vi "niWLAN - 80211abgnGeneration.vi"(0 "Rx Measurements Settings":T1={"Standard"=3, "Channel Bandwidth (Hz)"=40000000.0, "Idle Interval (s)"=400000.0, "MCS Index"=7, "80211n PLCP Frame Format"=0, "Payload Data Length (bytes)"=1024, "OFDM Data Rate (Mbps)"=0, "DSSS Data Rate (Mbps)"=0, "HW Settings"=[{"Carrier Frequency(Hz)"=5190000000.0, "power Level(dBm)"=[-10.0, -12.0, -14.0, -16.0, -18.0, -20.0, -22.0, -24.0, -26.0, -28.0, -30.0, -32.0, -34.0, -36.0, -38.0, -40.0, -42.0, -44.0, -46.0, -48.0, -50.0, -52.0, -54.0, -56.0, -58.0, -60.0, -62.0, -64.0, -66.0, -68.0, -70.0, -72.0, -74.0, -76.0, -78.0, -80.0, -82.0, -84.0], "power Level(milli-dBm)"=[-10000, -12000, -14000, -16000, -18000, -20000, -22000, -24000, -26000, -28000, -30000, -32000, -34000, -36000, -38000, -40000, -42000, -44000, -46000, -48000, -50000, -52000, -54000, -56000, -58000, -60000, -62000, -64000, -66000, -68000, -70000, -72000, -74000, -76000, -78000, -80000, -82000, -84000]}, {"Carrier Frequency(Hz)"=5230000000.0, "power Level(dBm)"=[-10.0, -12.0, -14.0, -16.0, -18.0, -20.0, -22.0, -24.0, -26.0, -28.0, -30.0, -32.0, -34.0, -36.0, -38.0, -40.0, -42.0, -44.0, -46.0, -48.0, -50.0, -52.0, -54.0, -56.0, -58.0, -60.0, -62.0, -64.0, -66.0, -68.0, -70.0, -72.0, -74.0, -76.0, -78.0, -80.0, -82.0, -84.0], "power Level(milli-dBm)"=[-10000, -12000, -14000, -16000, -18000, -20000, -22000, -24000, -26000, -28000, -30000, -32000, -34000, -36000, -38000, -40000, -42000, -44000, -46000, -48000, -50000, -52000, -54000, -56000, -58000, -60000, -62000, -64000, -66000, -68000, -70000, -72000, -74000, -76000, -78000, -80000, -82000, -84000]}, {"Carrier Frequency(Hz)"=5310000000.0, "power Level(dBm)"=[-10.0, -12.0, -14.0, -16.0, -18.0, -20.0, -22.0, -24.0, -26.0, -28.0, -30.0, -32.0, -34.0, -36.0, -38.0, -40.0, -42.0, -44.0, -46.0, -48.0, -50.0, -52.0, -54.0, -56.0, -58.0, -60.0, -62.0, -64.0, -66.0, -68.0, -70.0, -72.0, -74.0, -76.0, -78.0, -80.0, -82.0, -84.0], "power Level(milli-dBm)"=[-10000, -12000, -14000, -16000, -18000, -20000, -22000, -24000, -26000, -28000, -30000, -32000, -34000, -36000, -38000, -40000, -42000, -44000, -46000, -48000, -50000, -52000, -54000, -56000, -58000, -60000, -62000, -64000, -66000, -68000, -70000, -72000, -74000, -76000, -78000, -80000, -82000, -84000]}, {"Carrier Frequency(Hz)"=5510000000.0, "power Level(dBm)"=[-10.0, -12.0, -14.0, -16.0, -18.0, -20.0, -22.0, -24.0, -26.0, -28.0, -30.0, -32.0, -34.0, -36.0, -38.0, -40.0, -42.0, -44.0, -46.0, -48.0, -50.0, -52.0, -54.0, -56.0, -58.0, -60.0, -62.0, -64.0, -66.0, -68.0, -70.0, -72.0, -74.0, -76.0, -78.0, -80.0, -82.0, -84.0], "power Level(milli-dBm)"=[-10000, -12000, -14000, -16000, -18000, -20000, -22000, -24000, -26000, -28000, -30000, -32000, -34000, -36000, -38000, -40000, -42000, -44000, -46000, -48000, -50000, -52000, -54000, -56000, -58000, -60000, -62000, -64000, -66000, -68000, -70000, -72000, -74000, -76000, -78000, -80000, -82000, -84000]}, {"Carrier Frequency(Hz)"=5630000000.0, "power Level(dBm)"=[-10.0, -12.0, -14.0, -16.0, -18.0, -20.0, -22.0, -24.0, -26.0, -28.0, -30.0, -32.0, -34.0, -36.0, -38.0, -40.0, -42.0, -44.0, -46.0, -48.0, -50.0, -52.0, -54.0, -56.0, -58.0, -60.0, -62.0, -64.0, -66.0, -68.0, -70.0, -72.0, -74.0, -76.0, -78.0, -80.0, -82.0, -84.0], "power Level(milli-dBm)"=[-10000, -12000, -14000, -16000, -18000, -20000, -22000, -24000, -26000, -28000, -30000, -32000, -34000, -36000, -38000, -40000, -42000, -44000, -46000, -48000, -50000, -52000, -54000, -56000, -58000, -60000, -62000, -64000, -66000, -68000, -70000, -72000, -74000, -76000, -78000, -80000, -82000, -84000]}, {"Carrier Frequency(Hz)"=5670000000.0, "power Level(dBm)"=[-10.0, -12.0, -14.0, -16.0, -18.0, -20.0, -22.0, -24.0, -26.0, -28.0, -30.0, -32.0, -34.0, -36.0, -38.0, -40.0, -42.0, -44.0, -46.0, -48.0, -50.0, -52.0, -54.0, -56.0, -58.0, -60.0, -62.0, -64.0, -66.0, -68.0, -70.0, -72.0, -74.0, -76.0, -78.0, -80.0, -82.0, -84.0], "power Level(milli-dBm)"=[-10000, -12000, -14000, -16000, -18000, -20000, -22000, -24000, -26000, -28000, -30000, -32000, -34000, -36000, -38000, -40000, -42000, -44000, -46000, -48000, -50000, -52000, -54000, -56000, -58000, -60000, -62000, -64000, -66000, -68000, -70000, -72000, -74000, -76000, -78000, -80000, -82000, -84000]}, {"Carrier Frequency(Hz)"=5755000000.0, "power Level(dBm)"=[-10.0, -12.0, -14.0, -16.0, -18.0, -20.0, -22.0, -24.0, -26.0, -28.0, -30.0, -32.0, -34.0, -36.0, -38.0, -40.0, -42.0, -44.0, -46.0, -48.0, -50.0, -52.0, -54.0, -56.0, -58.0, -60.0, -62.0, -64.0, -66.0, -68.0, -70.0, -72.0, -74.0, -76.0, -78.0, -80.0, -82.0, -84.0], "power Level(milli-dBm)"=[-10000, -12000, -14000, -16000, -18000, -20000, -22000, -24000, -26000, -28000, -30000, -32000, -34000, -36000, -38000, -40000, -42000, -44000, -46000, -48000, -50000, -52000, -54000, -56000, -58000, -60000, -62000, -64000, -66000, -68000, -70000, -72000, -74000, -76000, -78000, -80000, -82000, -84000]}, {"Carrier Frequency(Hz)"=5795000000.0, "power Level(dBm)"=[-10.0, -12.0, -14.0, -16.0, -18.0, -20.0, -22.0, -24.0, -26.0, -28.0, -30.0, -32.0, -34.0, -36.0, -38.0, -40.0, -42.0, -44.0, -46.0, -48.0, -50.0, -52.0, -54.0, -56.0, -58.0, -60.0, -62.0, -64.0, -66.0, -68.0, -70.0, -72.0, -74.0, -76.0, -78.0, -80.0, -82.0, -84.0], "power Level(milli-dBm)"=[-10000, -12000, -14000, -16000, -18000, -20000, -22000, -24000, -26000, -28000, -30000, -32000, -34000, -36000, -38000, -40000, -42000, -44000, -46000, -48000, -50000, -52000, -54000, -56000, -58000, -60000, -62000, -64000, -66000, -68000, -70000, -72000, -74000, -76000, -78000, -80000, -82000, -84000]}]} {"DSSS Data Rate (Mbps)" items=["1", "2", "5.5 CCK", "5.5 PBCC", "11 CCK", "11 PBCC", "22", "33"]; "OFDM Data Rate (Mbps)" items=["6", "9", "12", "18", "24", "36", "48", "54"]; "80211n PLCP Frame Format" items=["Mixed Format", "Greenfield Format"]; "Standard" items=["80211A/G/J/P OFDM", "80211B/G DSSS", "80211G DSSSOFDM", "80211N MIMOOFDM", "80211AC MIMOOFDM"]}, 7 "Address String":string="00:90:4C:C5:12:38", 11 "error in":errorcluster={"status"=FALSE, "code"=373404, "source"="niRFSG Check Generation Status.vi<ERR>DSP overflow detected. Output waveform was clipped. Reduce the Arb Pre Filter Gain to eliminate overflow.\n\n "}) -> (4 "actual headroom (dB)":dbl, 6 "Waveforms":cluster{"t0":dbl, "dt":dbl, "Y":cdb[]}[](array[cluster])=[{"t0"=0.0, "dt"=1.25e-08, "Y"=[0.0+0.0i, 0.0+0.0i, 0.0+0.0i, 0.0+0.0i, 0.0+0.0i, 0.0+0.0i, 0.0+0.0i, 0.0+0.0i, 0.0+0.0i, 0.0+0.0i, 0.0+0.0i, 0.0+0.0i, 0.0+0.0i, 0.0+0.0i, 0.0+0.0i, 0.0+0.0i, 0.0+0.0i, 0.0+0.0i, 0.0+0.0i, 0.0+0.0i, 0.0+0.0i, 0.0+0.0i, 0.0+0.0i, 0.0+0.0i, 0.0+0.0i, 0.0+0.0i, 0.0+0.0i, 0.0+0.0i, 0.0+0.0i, 0.0+0.0i, 0.0+0.0i, 0.0+0.0i, 0.0+0.0i, 0.0+0.0i, 0.0+0.0i, 0.0+0.0i, 0.0+0.0i, 0.0+0.0i, 0.0+0.0i, 0.0+0.0i, 0.0+0.0i, 0.0+0.0i, 0.0+0.0i, 0.0+0.0i, 0.0+0.0i, 0.0+0.0i, 0.0+0.0i, 0.0+0.0i, 0.0+0.0i, 0.0+0.0i, 0.0+0.0i, 0.0+0.0i, 0.0+0.0i, 0.0+0.0i, 0.0+0.0i, 0.0+0.0i, 0.0+0.0i, 0.0+0.0i, 0.0+0.0i, 0.0+0.0i, 0.0+0.0i, 0.0+0.0i, 0.0+0.0i, 0.0+0.0i, 0.0+0.0i, 0.0+0.0i, 0.0+0.0i, 0.0+0.0i, 0.0+0.0i, 0.0+0.0i, 0.0+0.0i, 0.0+0.0i, 0.0+0.0i, 0.0+0.0i, 0.0+0.0i, 0.0+0.0i, 0.0+0.0i, 0.0+0.0i, 0.0+0.0i, 0.0+0.0i, 0.0+0.0i, 0.0+0.0i, 0.0+0.0i, 0.0+0.0i, 0.0+0.0i, 0.0+0.0i, 0.0+0.0i, 0.0+0.0i, 0.0+0.0i, 0.0+0.0i, 0.0+0.0i, 0.0+0.0i, 0.0+0.0i, 0.0+0.0i, 0.0+0.0i, 0.0+0.0i, 0.0+0.0i, 0.0+0.0i, 0.0+0.0i, 0.0+0.0i, 0.0+0.0i, 0.0+0.0i, 0.0+0.0i, 0.0+0.0i, 0.0+0.0i, 0.0+0.0i, 0.0+0.0i, 0.0+0.0i, 0.0+0.0i, 0.0+0.0i, 0.0+0.0i, 0.0+0.0i, 0.0+0.0i, 0.0+0.0i, 0.0+0.0i, 0.0+0.0i, 0.0+0.0i, 0.0+0.0i, 0.0+0.0i, 0.0+0.0i, 0.0+0.0i, 0.0+0.0i, 0.0+0.0i, 0.0+0.0i, 0.0+0.0i, 0.0+0.0i, 0.0+0.0i, 0.0+0.0i, 0.0+0.0i, 0.0+0.0i, 0.0+0.0i, 0.0+0.0i, 0.0+0.0i, 0.0+0.0i, 0.0+0.0i, 0.0+0.0i, 0.0+0.0i, 0.0+0.0i, 0.0+0.0i, 0.0+0.0i, 0.0+0.0i, 0.0+0.0i, 0.0+0.0i, 0.0+0.0i, 0.0+0.0i, 0.0+0.0i, 0.0+0.0i, 0.0+0.0i, 0.0+0.0i, 0.0+0.0i, 0.0+0.0i, 0.0+0.0i, 0.0+0.0i, 0.0+0.0i, 0.0+0.0i, 0.0+0.0i, 0.0+0.0i, 0.0+0.0i, 0.0+0.0i, 0.0+0.0i, 0.0+0.0i, 0.0+0.0i, 0.0+0.0i, 0.0+0.0i, 0.0+0.0i, 0.0+0.0i, 0.0+0.0i, 0.0+0.0i, 0.0+0.0i, 0.0+0.0i, 0.0+0.0i, 0.0+0.0i, 0.0+0.0i, 0.0+0.0i, 0.0+0.0i, 0.0+0.0i, 0.0+0.0i, 0.0+0.0i, 0.0+0.0i, 0.0+0.0i, 0.0+0.0i, 0.0+0.0i, 0.0+0.0i, 0.0+0.0i, 0.0+0.0i, 0.0+0.0i, 0.0+0.0i, 0.0+0.0i, 0.0+0.0i, 0.0+0.0i, 0.0+0.0i, 0.0+0.0i, 0.0+0.0i, 0.0+0.0i, 0.0+0.0i, 0.0+0.0i, 0.0+0.0i, 0.0+0.0i, 0.0+0.0i, 0.0+0.0i, 0.0+0.0i, 0.0+0.0i, 0.0+0.0i, 0.0+0.0i, 0.0+0.0i, 0.0+0.0i, 0.0+0.0i, 0.0+0.0i, 0.0+0.0i, 0.0+0.0i, 0.0+0.0i, 0.0+0.0i, 0.0+0.0i, 0.0+0.0i, 0.0+0.0i, 0.0+0.0i, 0.0+0.0i, 0.0+0.0i, 0.0+0.0i, 0.0+0.0i, 0.0+0.0i, 0.0+0.0i, 0.0+0.0i, 0.0+0.0i, 0.0+0.0i, 0.0+0.0i, 0.0+0.0i, 0.0+0.0i, 0.0+0.0i, 0.0+0.0i, 0.0+0.0i, 0.0+0.0i, 0.0+0.0i, 0.0+0.0i, 0.0+0.0i, 0.0+0.0i, 0.0+0.0i, 0.0+0.0i, 0.0+0.0i, 0.0+0.0i, 0.0+0.0i, 0.0+0.0i, 0.0+0.0i, 0.0+0.0i, 0.0+0.0i, 0.0+0.0i, 0.0+0.0i, 0.0+0.0i, 0.0+0.0i, 0.0+0.0i, 0.0+0.0i, 0.0+0.0i, 0.0+0.0i, 0.0+0.0i, 0.0+0.0i, 0.0+0.0i, 0.0+0.0i, 0.0+0.0i, 0.0+0.0i, 0.0+0.0i, 0.0+0.0i, 0.0+0.0i, 0.0+0.0i, 0.0+0.0i, 0.0+0.0i, 0.0+0.0i, 0.0+0.0i, 0.0+0.0i, 0.0+0.0i, 0.0+0.0i, 0.0+0.0i, 0.0+0.0i, 0.0+0.0i, 0.0+0.0i, 0.0+0.0i, 0.0+0.0i, 0.0+0.0i, 0.0+0.0i, 0.0+0.0i, 0.0+0.0i, 0.0+0.0i, 0.0+0.0i, 0.0+0.0i, 0.0+0.0i, 0.0+0.0i, 0.0+0.0i, 0.0+0.0i, 0.0+0.0i, 0.0+0.0i, 0.0+0.0i, 0.0+0.0i, 0.0+0.0i, 0.0+0.0i, 0.0+0.0i, 0.0+0.0i, 0.0+0.0i, 0.0+0.0i, 0.0+0.0i, 0.0+0.0i, 0.0+0.0i, 0.0+0.0i, 0.0+0.0i, 0.0+0.0i, 0.0+0.0i, 0.0+0.0i, 0.0+0.0i, 0.0+0.0i, 0.0+0.0i, 0.0+0.0i, 0.0+0.0i, 0.0+0.0i, 0.0+0.0i, 0.0+0.0i, 0.0+0.0i, 0.0+0.0i, 0.0+0.0i, 0.0+0.0i, 0.0+0.0i, 0.0+0.0i, 0.0+0.0i, 0.0+0.0i, 0.0+0.0i, 0.0+0.0i, 0.0+0.0i, 0.0+0.0i, 0.0+0.0i, 0.0+0.0i, 0.0+0.0i, 0.0+0.0i, 0.0+0.0i, 0.0+0.0i, 0.0+0.0i, 0.0+0.0i, 0.0+0.0i, 0.0+0.0i, 0.0+0.0i, 0.0+0.0i, 0.0+0.0i, 0.0+0.0i, 0.0+0.0i, 0.0+0.0i, 0.0+0.0i, 0.0+0.0i, 0.0+0.0i, 0.0+0.0i, 0.0+0.0i, 0.0+0.0i, 0.0+0.0i, 0.0+0.0i, 0.0+0.0i, 0.0+0.0i, 0.0+0.0i, 0.0+0.0i, 0.0+0.0i, 0.0+0.0i, 0.0+0.0i, 0.0+0.0i, 0.0+0.0i, 0.0+0.0i, 0.0+0.0i, 0.0+0.0i, 0.0+0.0i, 0.0+0.0i, 0.0+0.0i, 0.0+0.0i, 0.0+0.0i, 0.0+0.0i, 0.0+0.0i, 0.0+0.0i, 0.0+0.0i, 0.0+0.0i, 0.0+0.0i, 0.0+0.0i, 0.0+0.0i, 0.0+0.0i, 0.0+0.0i, 0.0+0.0i, 0.0+0.0i, 0.0+0.0i, 0.0+0.0i, 0.0+0.0i, 0.0+0.0i, 0.0+0.0i, 0.0+0.0i, 0.0+0.0i, 0.0+0.0i, 0.0+0.0i, 0.0+0.0i, 0.0+0.0i, 0.0+0.0i, 0.0+0.0i, 0.0+0.0i, 0.0+0.0i, 0.0+0.0i, 0.0+0.0i, 0.0+0.0i, 0.0+0.0i, 0.0+0.0i, 0.0+0.0i, 0.0+0.0i, 0.0+0.0i, 0.0+0.0i, 0.0+0.0i, 0.0+0.0i, 0.0+0.0i, 0.0+0.0i, 0.0+0.0i, 0.0+0.0i, 0.0+0.0i, 0.0+0.0i, 0.0+0.0i, 0.0+0.0i, 0.0+0.0i, 0.0+0.0i, 0.0+0.0i, 0.0+0.0i, 0.0+0.0i, 0.0+0.0i, 0.0+0.0i, 0.0+0.0i, 0.0+0.0i, 0.0+0.0i, 0.0+0.0i, 0.0+0.0i, 0.0+0.0i, 0.0+0.0i, 0.0+0.0i, 0.0+0.0i, 0.0+0.0i, 0.0+0.0i, 0.0+0.0i, 0.0+0.0i, 0.0+0.0i, 0.0+0.0i, 0.0+0.0i, 0.0+0.0i, 0.0+0.0i, 0.0+0.0i, 0.0+0.0i, 0.0+0.0i, 0.0+0.0i, 0.0+0.0i, 0.0+0.0i, 0.0+0.0i, 0.0+0.0i, 0.0+0.0i, 0.0+0.0i, 0.0+0.0i, 0.0+0.0i, 0.0+0.0i, 0.0+0.0i, 0.0+0.0i, 0.0+0.0i, 0.0+0.0i, 0.0+0.0i, 0.0+0.0i, 0.0+0.0i, 0.0+0.0i, 0.0+0.0i, 0.0+0.0i, 0.0+0.0i, 0.0+0.0i, 0.0+0.0i, 0.0+0.0i, 0.0+0.0i, 0.0+0.0i, 0.0+0.0i, 0.0+0.0i, 0.0+0.0i, 0.0+0.0i, 0.0+0.0i, 0.0+0.0i, 0.0+0.0i, 0.0+0.0i, 0.0+0.0i, 0.0+0.0i, 0.0+0.0i, 0.0+0.0i, 0.0+0.0i, 0.0+0.0i, 0.0+0.0i, 0.0+0.0i, 0.0+0.0i, 0.0+0.0i, 0.0+0.0i, 0.0+0.0i, 0.0+0.0i, 0.0+0.0i, 0.0+0.0i, 0.0+0.0i, 0.0+0.0i, 0.0+0.0i, 0.0+0.0i, 0.0+0.0i, 0.0+0.0i, 0.0+0.0i, 0.0+0.0i, 0.0+0.0i, 0.0+0.0i, 0.0+0.0i, 0.0+0.0i, 0.0+0.0i, 0.0+0.0i, 0.0+0.0i, 0.0+0.0i, 0.0+0.0i, 0.0+0.0i, 0.0+0.0i, 0.0+0.0i, 0.0+0.0i, 0.0+0.0i, 0.0+0.0i, 0.0+0.0i, 0.0+0.0i, 0.0+0.0i, 0.0+0.0i, 0.0+0.0i, 0.0+0.0i, 0.0+0.0i, 0.0+0.0i, 0.0+0.0i, 0.0+0.0i, 0.0+0.0i, 0.0+0.0i, 0.0+0.0i, 0.0+0.0i, 0.0+0.0i, 0.0+0.0i, 0.0+0.0i, 0.0+0.0i, 0.0+0.0i, 0.0+0.0i, 0.0+0.0i, 0.0+0.0i, 0.0+0.0i, 0.0+0.0i, 0.0+0.0i, 0.0+0.0i, 0.0+0.0i, 0.0+0.0i, 0.0+0.0i, 0.0+0.0i, 0.0+0.0i, 0.0+0.0i, 0.0+0.0i, 0.0+0.0i, 0.0+0.0i, 0.0+0.0i, 0.0+0.0i, 0.0+0.0i, 0.0+0.0i, 0.0+0.0i, 0.0+0.0i, 0.0+0.0i, 0.0+0.0i, 0.0+0.0i, 0.0+0.0i, 0.0+0.0i, 0.0+0.0i, 0.0+0.0i, 0.0+0.0i, 0.0+0.0i, 0.0+0.0i, 0.0+0.0i, 0.0+0.0i, 0.0+0.0i, 0.0+0.0i, 0.0+0.0i, 0.0+0.0i, 0.0+0.0i, 0.0+0.0i, 0.0+0.0i, 0.0+0.0i, 0.0+0.0i, 0.0+0.0i, 0.0+0.0i, 0.0+0.0i, 0.0+0.0i, 0.0+0.0i, 0.0+0.0i, 0.0+0.0i, 0.0+0.0i, 0.0+0.0i, 0.0+0.0i, 0.0+0.0i, 0.0+0.0i, 0.0+0.0i, 0.0+0.0i, 0.0+0.0i, 0.0+0.0i, 0.0+0.0i, 0.0+0.0i, 0.0+0.0i, 0.0+0.0i, 0.0+0.0i, 0.0+0.0i, 0.0+0.0i, 0.0+0.0i, 0.0+0.0i, 0.0+0.0i, 0.0+0.0i, 0.0+0.0i, 0.0+0.0i, 0.0+0.0i, 0.0+0.0i, 0.0+0.0i, 0.0+0.0i, 0.0+0.0i, 0.0+0.0i, 0.0+0.0i, 0.0+0.0i, 0.0+0.0i, 0.0+0.0i, 0.0+0.0i, 0.0+0.0i, 0.0+0.0i, 0.0+0.0i, 0.0+0.0i, 0.0+0.0i, 0.0+0.0i, 0.0+0.0i, 0.0+0.0i, 0.0+0.0i, 0.0+0.0i, 0.0+0.0i, 0.0+0.0i, 0.0+0.0i, 0.0+0.0i, 0.0+0.0i, 0.0+0.0i, 0.0+0.0i, 0.0+0.0i, 0.0+0.0i, 0.0+0.0i, 0.0+0.0i, 0.0+0.0i, 0.0+0.0i, 0.0+0.0i, 0.0+0.0i, 0.0+0.0i, 0.0+0.0i, 0.0+0.0i, 0.0+0.0i, 0.0+0.0i, 0.0+0.0i, 0.0+0.0i, 0.0+0.0i, 0.0+0.0i, 0.0+0.0i, 0.0+0.0i, 0.0+0.0i, 0.0+0.0i, 0.0+0.0i, 0.0+0.0i, 0.0+0.0i, 0.0+0.0i, 0.0+0.0i, 0.0+0.0i, 0.0+0.0i, 0.0+0.0i, 0.0+0.0i, 0.0+0.0i, 0.0+0.0i, 0.0+0.0i, 0.0+0.0i, 0.0+0.0i, 0.0+0.0i, 0.0+0.0i, 0.0+0.0i, 0.0+0.0i, 0.0+0.0i, 0.0+0.0i, 0.0+0.0i, 0.0+0.0i, 0.0+0.0i, 0.0+0.0i, 0.0+0.0i, 0.0+0.0i, 0.0+0.0i, 0.0+0.0i, 0.0+0.0i, 0.0+0.0i, 0.0+0.0i, 0.0+0.0i, 0.0+0.0i, 0.0+0.0i, 0.0+0.0i, 0.0+0.0i, 0.0+0.0i, 0.0+0.0i, 0.0+0.0i, 0.0+0.0i, 0.0+0.0i, 0.0+0.0i, 0.0+0.0i, 0.0+0.0i, 0.0+0.0i, 0.0+0.0i, 0.0+0.0i, 0.0+0.0i, 0.0+0.0i, 0.0+0.0i, 0.0+0.0i, 0.0+0.0i, 0.0+0.0i, 0.0+0.0i, 0.0+0.0i, 0.0+0.0i, 0.0+0.0i, 0.0+0.0i, 0.0+0.0i, 0.0+0.0i, 0.0+0.0i, 0.0+0.0i, 0.0+0.0i, 0.0+0.0i, 0.0+0.0i, 0.0+0.0i, 0.0+0.0i, 0.0+0.0i, 0.0+0.0i, 0.0+0.0i, 0.0+0.0i, 0.0+0.0i, 0.0+0.0i, 0.0+0.0i, 0.0+0.0i, 0.0+0.0i, 0.0+0.0i, 0.0+0.0i, 0.0+0.0i, 0.0+0.0i, 0.0+0.0i, 0.0+0.0i, 0.0+0.0i, 0.0+0.0i, 0.0+0.0i, 0.0+0.0i, 0.0+0.0i, 0.0+0.0i, 0.0+0.0i, 0.0+0.0i, 0.0+0.0i, 0.0+0.0i, 0.0+0.0i, 0.0+0.0i, 0.0+0.0i, 0.0+0.0i, 0.0+0.0i, 0.0+0.0i, 0.0+0.0i, 0.0+0.0i, 0.0+0.0i, 0.0+0.0i, 0.0+0.0i, 0.0+0.0i, 0.0+0.0i, 0.0+0.0i, 0.0+0.0i, 0.0+0.0i, 0.0+0.0i, 0.0+0.0i, 0.0+0.0i, 0.0+0.0i, 0.0+0.0i, 0.0+0.0i, 0.0+0.0i, 0.0+0.0i, 0.0+0.0i, 0.0+0.0i, 0.0+0.0i, 0.0+0.0i, 0.0+0.0i, 0.0+0.0i, 0.0+0.0i, 0.0+0.0i, 0.0+0.0i, 0.0+0.0i, 0.0+0.0i, 0.0+0.0i, 0.0+0.0i, 0.0+0.0i, 0.0+0.0i, 0.0+0.0i, 0.0+0.0i, 0.0+0.0i, 0.0+0.0i, 0.0+0.0i, 0.0+0.0i, 0.0+0.0i, 0.0+0.0i, 0.0+0.0i, 0.0+0.0i, 0.0+0.0i, 0.0+0.0i, 0.0+0.0i, 0.0+0.0i, 0.0+0.0i, 0.0+0.0i, 0.0+0.0i]}, ...(2 in all)], 8 "wfm Size in msec":i32=1, 10 "Size in Samples":i32[](array[numeric])=[10000000, 0], 14 "40M?":bool=TRUE, 15 "error out":errorcluster={"status"=FALSE, "code"=373404, "source"="niRFSG Check Generation Status.vi<ERR>DSP overflow detected. Output waveform was clipped. Reduce the Arb Pre Filter Gain to eliminate overflow.\n\n "})   [LabVIEW 2011]
uses:
  TV/RW/Includes/WLAN - TV - RW - INC - TV_Format_Rx.ctl
  <vilib>/RF Toolkits/WLAN/generation/controls/wlanG version control.ctl
  <vilib>/RF Toolkits/WLAN/generation/niWLANG Create Multiple Channel Waveform (IQ Complex Cluster).vi
  <vilib>/RF Toolkits/WLAN/generation/niWLANG Create Single Channel Waveform (IQ Complex Cluster).vi
  Program Files/National Instruments/LabVIEW 2011/resource/objmgr/niWLANGeneration.rc
panel:
  # "Hardware Configuration"
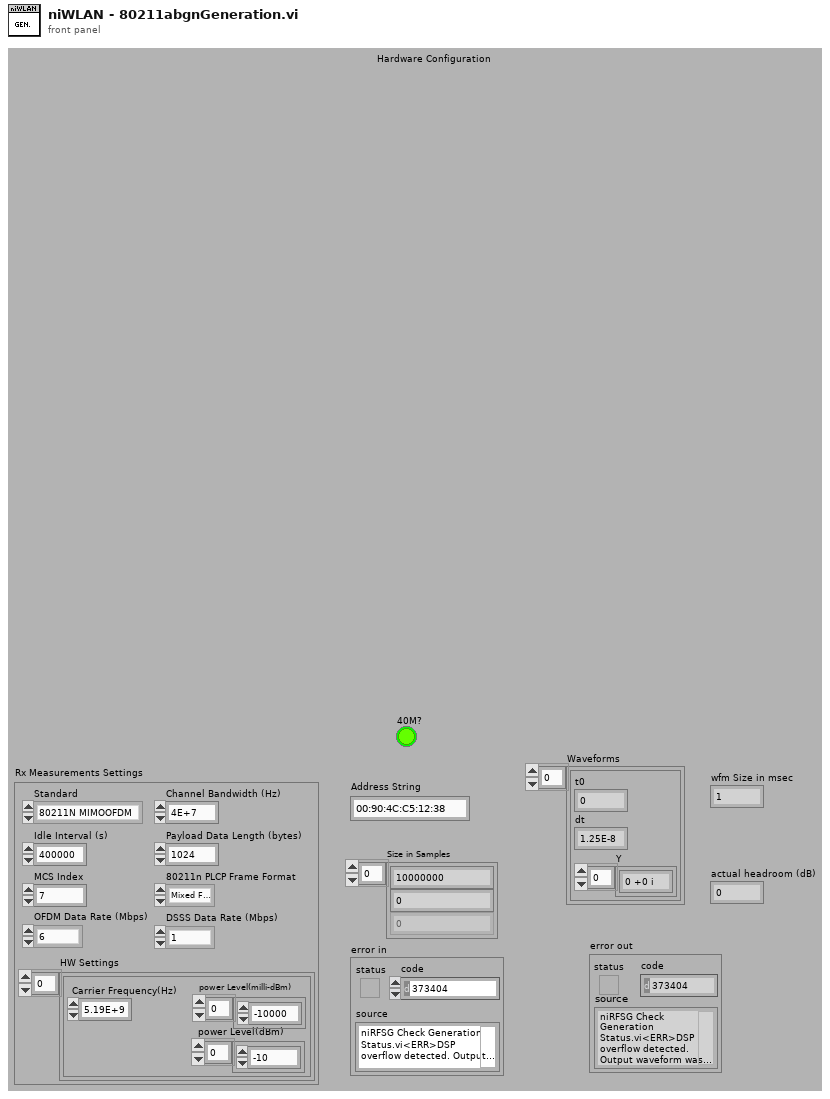
[diagram p1: front panel]
types:
  T1 = typedef "WLAN - TV - RW - INC - TV_Format_Rx.ctl" = cluster{"Standard":i32, "Channel Bandwidth (Hz)":dbl, "Idle Interval (s)":dbl, "MCS Index":i32, "80211n PLCP Frame Format":i32, "Payload Data Length (bytes)":i32, "OFDM Data Rate (Mbps)":i32, "DSSS Data Rate (Mbps)":i32, "HW Settings":cluster{"Carrier Frequency(Hz)":dbl, "power Level(dBm)":dbl[], "power Level(milli-dBm)":i32[]}[]}
  T2 = typedef "wlanG version control.ctl" = i32
  T3 = typedef "wlanv1_generation refnum.ctl" = refnum<k20>
  T4 = typedef "wlanv1_Generation Refnum.ctl" = refnum<k20>
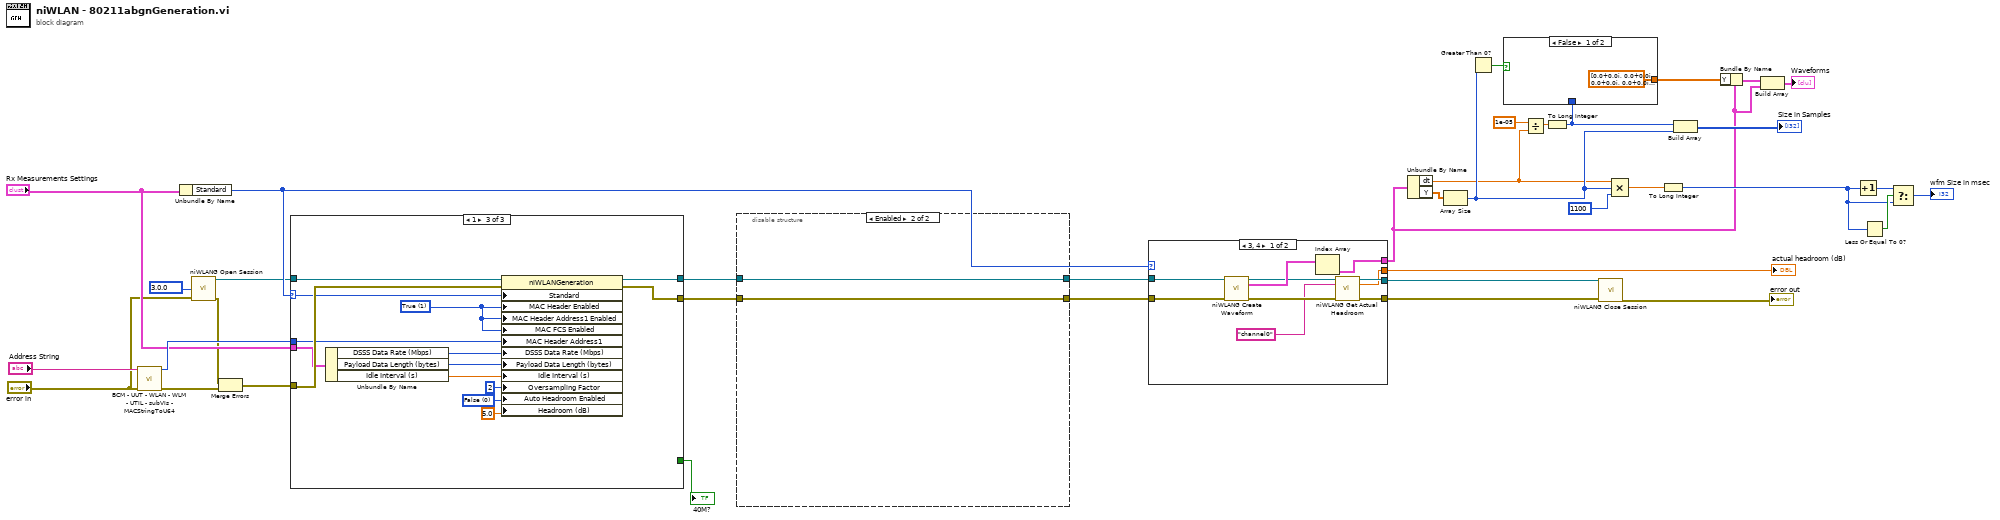
[diagram p0: block diagram]
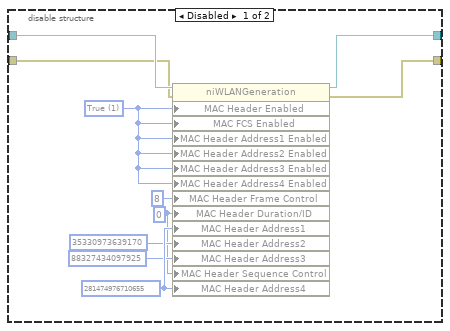
[diagram p2: hidden frame]
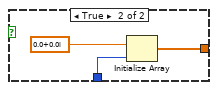
[diagram p3: hidden frame]
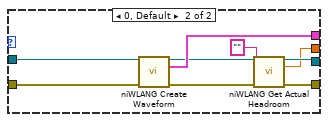
[diagram p4: hidden frame]
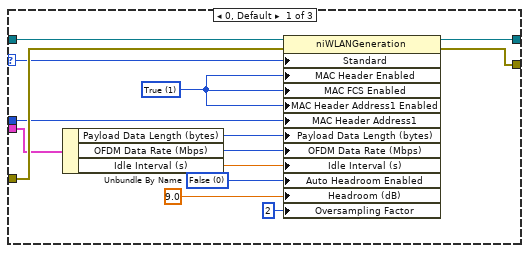
[diagram p5: hidden frame]
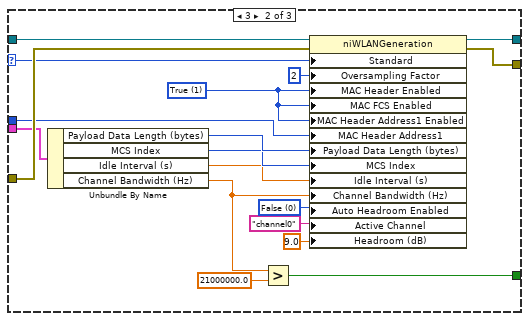
[diagram p6: hidden frame]
diagram:
  w29 = T2 30000 items=["1.0.0"=10000, "2.0.0"=20000, "3.0.0"=30000] ("toolkit compatibility version")
  n1 = call "BCM - UUT - WLAN - WLM - UTIL - subVIs - MACStringToU64.vi"("Address String"="Address String", "error in"="error in") -> ("Address U64"=w37:u64, "error out"=w26:errorcluster)  [unwired: 12 in]
  n2 = Unbundle By Name("Rx Measurements Settings") -> ("Standard"=w32:i32)
  n3 = call <vilib>:"niWLANG Open Session.vi"("toolkit compatibility version"=w29, "error in"="error in") -> ("niwlan generation session"=w30:T3, "error out"=w27:errorcluster)  [unwired: 11 in, 1 out]
  n4 = Merge Errors(w27, w26) -> (w25:errorcluster)
  n5 = case shown="1" w32 {
    selector: w32 -> [w46 w64 w79]
    tunnel: w30 -> [w51 w68 w83]
    tunnel: w25 -> [w50 w65 w82]
    tunnel: [w49 w67 w81] -> w4
    tunnel: [w48 w66 w80] -> w2
    tunnel: w37 -> [w40 w57 w74]
    tunnel: "Rx Measurements Settings" -> [w44 w61 w76]
    tunnel: [_ w53 _] -> w8
    frame 0, Default {
      w43 = 0 items=["False", "True"] ("Auto Headroom Enabled")
      w47 = 1 items=["False", "True"] ("MAC Header Enabled")
      n6 = Unbundle By Name(w44) -> ("Payload Data Length (bytes)"=w41:i32, "OFDM Data Rate (Mbps)"=w45:i32, "Idle Interval (s)"=w39:dbl)
      n7 = property class="niWLANGeneration"(reference=w51, error in=w50, "Standard"=w46, "MAC Header Enabled"=w47, "MAC FCS Enabled"=w47, "MAC Header Address1 Enabled"=w47, "MAC Header Address1"=w40, "Payload Data Length (bytes)"=w41, "OFDM Data Rate (Mbps)"=w45, "Idle Interval (s)"=w39, "Auto Headroom Enabled"=w43, "Headroom (dB)"=9.0, "Oversampling Factor"=2) -> (reference out=w49:T3, error out=w48:errorcluster)
    }
    frame 3 {
      w60 = 0 items=["False", "True"] ("Auto Headroom Enabled")
      w69 = 1 items=["False", "True"] ("MAC Header Enabled")
      n8 = Unbundle By Name(w61) -> ("Payload Data Length (bytes)"=w63:i32, "MCS Index"=w62:i32, "Idle Interval (s)"=w56:dbl, "Channel Bandwidth (Hz)"=w55:dbl)
      n9 = Greater?(x=w55, y=21000000.0) -> (0:w53:bool)
      n10 = property class="niWLANGeneration"(reference=w68, error in=w65, "Standard"=w64, "Oversampling Factor"=2, "MAC Header Enabled"=w69, "MAC FCS Enabled"=w69, "MAC Header Address1 Enabled"=w69, "MAC Header Address1"=w57, "Payload Data Length (bytes)"=w63, "MCS Index"=w62, "Idle Interval (s)"=w56, "Channel Bandwidth (Hz)"=w55, "Auto Headroom Enabled"=w60, "Active Channel"="channel0", "Headroom (dB)"=9.0) -> (reference out=w67:T3, error out=w66:errorcluster)
    }
    frame 1 {
      w71 = 0 items=["False", "True"] ("Auto Headroom Enabled")
      w78 = 1 items=["False", "True"] ("OFDM Demod Enabled")
      n11 = Unbundle By Name(w76) -> ("DSSS Data Rate (Mbps)"=w77:i32, "Payload Data Length (bytes)"=w75:i32, "Idle Interval (s)"=w73:dbl)
      n12 = property class="niWLANGeneration"(reference=w83, error in=w82, "Standard"=w79, "MAC Header Enabled"=w78, "MAC Header Address1 Enabled"=w78, "MAC FCS Enabled"=w78, "MAC Header Address1"=w74, "DSSS Data Rate (Mbps)"=w77, "Payload Data Length (bytes)"=w75, "Idle Interval (s)"=w73, "Oversampling Factor"=2, "Auto Headroom Enabled"=w71, "Headroom (dB)"=5.0) -> (reference out=w81:T3, error out=w80:errorcluster)
    }
  }
  "40M?" <- w8
  n13 = disable-structure shown="Enabled" {
    disable-tunnel: w4 -> [w93 w95]
    disable-tunnel: [w92 w95] -> w3
    disable-tunnel: w2 -> [w91 w94]
    disable-tunnel: [w90 w94] -> w1
    frame Disabled {
      w87 = i64 281474976710655 ("MAC Header Address4")
      w84 = 0 ("MAC Header Frame Control")
      w89 = 1 items=["False", "True"] ("MAC Header Enabled")
      n14 = property class="niWLANGeneration"(reference=w93, error in=w91, "MAC Header Enabled"=w89, "MAC FCS Enabled"=w89, "MAC Header Address1 Enabled"=w89, "MAC Header Address2 Enabled"=w89, "MAC Header Address3 Enabled"=w89, "MAC Header Address4 Enabled"=w89, "MAC Header Frame Control"=8, "MAC Header Duration/ID"=w84, "MAC Header Address1"=w87, "MAC Header Address2"=i64 35330973639170 ("MAC Header Address4"), "MAC Header Address3"=i64 88327434097925 ("MAC Header Address4"), "MAC Header Sequence Control"=w84, "MAC Header Address4"=w87) -> (reference out=w92:T3, error out=w90:errorcluster)
    }
    frame Enabled {
    }
  }
  n15 = case shown="3, 4" w32 {
    tunnel: [w100 w110] -> w22
    tunnel: w3 -> [w104 w114]
    tunnel: w1 -> [w105 w113]
    tunnel: [w98 w109] -> w24
    tunnel: [w102 w112] -> w9
    tunnel: [w96 w107] -> w21
    frame 3, 4 {
      n16 = call-poly <vilib>:"niWLANG Create Waveform.vi"("niwlan generation session"=w104, "error in"=w105) -> ("niwlan generation session out"=w101:T3, "output waveform"=w103:cluster{"t0":dbl, "dt":dbl, "Y":cdb[]}[], "error out"=w99:errorcluster)  [unwired: 10 in, 1 out]
      n17 = Index Array(array=w103) -> (element=w102:cluster{"t0":dbl, "dt":dbl, "Y":cdb[]})  [unwired: 1 in]
      n18 = call <vilib>:"niWLANG Get Actual Headroom.vi"("niwlan generation session"=w101, "active channel"="channel0", "error in"=w99) -> ("niwlan generation session out"=w100:T4, "actual headroom (dB)"=w96:dbl, "error out"=w98:errorcluster)  [unwired: 10 in]
    }
    frame 0, Default {
      n19 = call-poly <vilib>:"niWLANG Create Waveform.vi"("niwlan generation session"=w114, "error in"=w113) -> ("niwlan generation session out"=w111:T3, "output waveform"=w112:cluster{"t0":dbl, "dt":dbl, "Y":cdb[]}, "error out"=w108:errorcluster)  [unwired: 10 in, 1 out]
      n20 = call <vilib>:"niWLANG Get Actual Headroom.vi"("niwlan generation session"=w111, "active channel"="", "error in"=w108) -> ("niwlan generation session out"=w110:T4, "actual headroom (dB)"=w107:dbl, "error out"=w109:errorcluster)  [unwired: 10 in]
    }
  }
  "actual headroom (dB)" <- w21
  n21 = Unbundle By Name(w9) -> ("dt"=w5:dbl, "Y"=w35:cdb[])
  n22 = Array Size(array=w35) -> (size(s)=w7:i32)
  n23 = Greater Than 0?(x=w7) -> (x > 0?=w6:bool)
  n24 = Divide(x=1e-05, y=w5) -> (x/y=w15:dbl)
  n25 = To Long Integer(number=w15) -> (32bit integer=w13:i32)
  n26 = case shown="False" w6 {
    tunnel: [cdb[] [0.0+0.0i, 0.0+0.0i, 0.0+0.0i, 0.0+0.0i, 0.0+0.0i, 0.0+0.0i, 0.0+0.0i, 0.0+0.0i, 0.0+0.0i, 0.0+0.0i, 0.0+0.0i, 0.0+0.0i, 0.0+0.0i, 0.0+0.0i, 0.0+0.0i, 0.0+0.0i, 0.0+0.0i, 0.0+0.0i, 0.0+0.0i, 0.0+0.0i, 0.0+0.0i, 0.0+0.0i, 0.0+0.0i, 0.0+0.0i, 0.0+0.0i, 0.0+0.0i, 0.0+0.0i, 0.0+0.0i, 0.0+0.0i, 0.0+0.0i, 0.0+0.0i, 0.0+0.0i, 0.0+0.0i, 0.0+0.0i, 0.0+0.0i, 0.0+0.0i, 0.0+0.0i, 0.0+0.0i, 0.0+0.0i, 0.0+0.0i, 0.0+0.0i, 0.0+0.0i, 0.0+0.0i, 0.0+0.0i, 0.0+0.0i, 0.0+0.0i, 0.0+0.0i, 0.0+0.0i, 0.0+0.0i, 0.0+0.0i, 0.0+0.0i, 0.0+0.0i, 0.0+0.0i, 0.0+0.0i, 0.0+0.0i, 0.0+0.0i, 0.0+0.0i, 0.0+0.0i, 0.0+0.0i, 0.0+0.0i, 0.0+0.0i, 0.0+0.0i, 0.0+0.0i, 0.0+0.0i, 0.0+0.0i, 0.0+0.0i, 0.0+0.0i, 0.0+0.0i, 0.0+0.0i, 0.0+0.0i, 0.0+0.0i, 0.0+0.0i, 0.0+0.0i, 0.0+0.0i, 0.0+0.0i, 0.0+0.0i, 0.0+0.0i, 0.0+0.0i, 0.0+0.0i, 0.0+0.0i, 0.0+0.0i, 0.0+0.0i, 0.0+0.0i, 0.0+0.0i, 0.0+0.0i, 0.0+0.0i, 0.0+0.0i, 0.0+0.0i, 0.0+0.0i, 0.0+0.0i, 0.0+0.0i, 0.0+0.0i, 0.0+0.0i, 0.0+0.0i, 0.0+0.0i, 0.0+0.0i, 0.0+0.0i, 0.0+0.0i, 0.0+0.0i, 0.0+0.0i, 0.0+0.0i] w117] -> w14
    tunnel: w13 -> [_ w116]
    frame False {
    }
    frame True {
      n27 = Initialize Array(cdb 0.0+0.0i ("element"), w116) -> (w117:cdb[])
    }
  }
  n28 = call <vilib>:"niWLANG Close Session.vi"("niwlan generation session"=w22, "error in"=w24) -> ("error out"=→"error out":errorcluster)  [unwired: 13 in]
  n29 = Compound Arithmetic op=MULTIPLY(w5, w7, 1100 ("y")) -> (w33:dbl)
  n30 = To Long Integer(number=w33) -> (32bit integer=w19:i32)
  n31 = Build Array(w13, w7) -> (→"Size in Samples":i32[])
  n32 = Bundle By Name(cluster=w9, "Y"=w14) -> (w12:cluster{"t0":dbl, "dt":dbl, "Y":cdb[]})
  n33 = Build Array(w12, w9) -> (→"Waveforms":cluster{"t0":dbl, "dt":dbl, "Y":cdb[]}[])
  n34 = Increment(x=w19) -> (x+1=w18:i32)
  n35 = Less Or Equal To 0?(x=w19) -> (x <= 0?=w20:bool)
  n36 = Select(t=w18, s=w20, f=w19) -> (s? t:f=→"wfm Size in msec":i32)
